vi "ExSubcenterStrip.vi"(2 "error in (no error)":errorcluster, 3 "Camera Handle":u32) -> (0 "error out":errorcluster, 1 "Camera Handle":u32)   [LabVIEW 2010]
panel:
  # "ExSubCenterStrip:\nThis sub-vi gets the camera dimensions\nand picks/programs the center strip/row \nas an ROI."
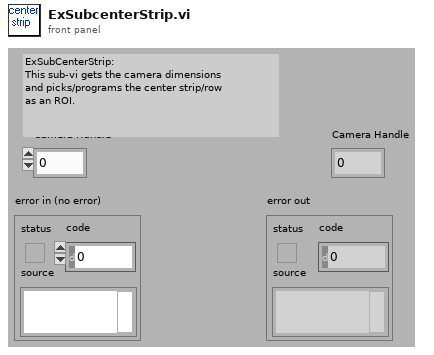
[diagram p1: front panel]
types:
  T1 = cluster{"X start":u32, "X end":u32, "X Binning/Grouping":u32, "Y start":u32, "Y end":u32, "Y Binning/Grouping":u32}
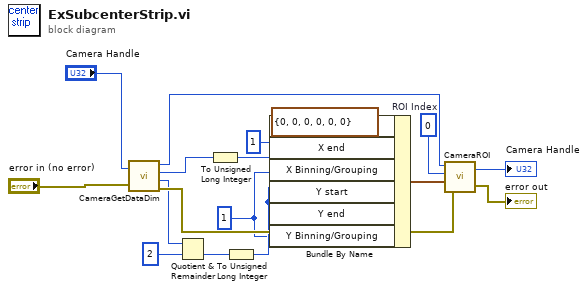
[diagram p0: block diagram]
diagram:
  w1 = u32 0  # ROI Index
  w4 = u32 1
  n1 = call <userlib>:"CameraGetDataDim.vi"("Camera Handle"="Camera Handle", "error in"="error in (no error)") -> ("Camera Handle"=w16:u32, "Xdim"=w13:u32, "Ydim"=w10:u32, "error out"=w14:errorcluster)
  n2 = Quotient & Remainder(x=w10, y=2) -> (floor(x/y)=w8:u32)  [unwired: 1 out]
  n3 = To Unsigned Long Integer(number=w13) -> (unsigned 32bit integer=w6:u32)
  n4 = To Unsigned Long Integer(number=w8) -> (unsigned 32bit integer=w5:u32)
  n5 = Bundle By Name(cluster=T1 {"X start"=0, "X end"=0, "X Binning/Grouping"=0, "Y start"=0, "Y end"=0, "Y Binning/Grouping"=0} ("ROI Params"), "X start"=u32 1, "X end"=w6, "X Binning/Grouping"=w4, "Y start"=w5, "Y end"=w5, "Y Binning/Grouping"=w4) -> (w3:T1)
  n6 = call <userlib>:"CameraROI.vi"("error in"=w14, "ROI Params"=w3, "ROI Index"=w1, "Camera Handle"=w16) -> ("error out"=→"error out":errorcluster, "Camera Handle"=→"Camera Handle":u32)
